vi "EXCEL TRIALS.vi"() -> ()   [LabVIEW 2021]
panel:
  out "PATH OUT":path
  in  "WRITE DATA INPUT":string
  out "READ RESPONSE":string
  in  "Enum":enum16{"READ", "WRITE"}(ring)
  in  "CLOSE/OPEN":bool
  in  "RANGE":string
  in  "Excel._Worksheet":refnum<k7>
  in  "SHEET":string
  in  "Stop":bool
  out "error out":errorcluster
  in  "error in":errorcluster
  in  "Excel._Application":refnum<k7>
  in  "PATH IN":path
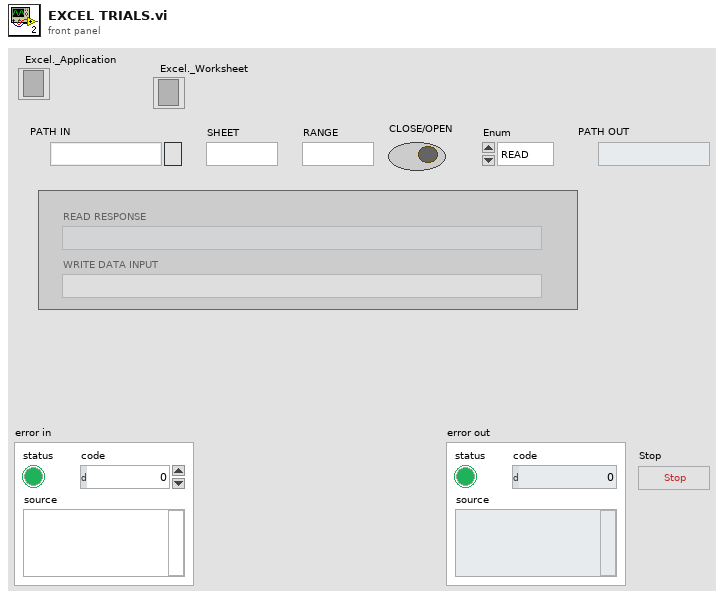
[diagram p1: front panel]
types:
  T1 = enum8{"Enabled", "Disabled", "Disabled and Grayed Out"}
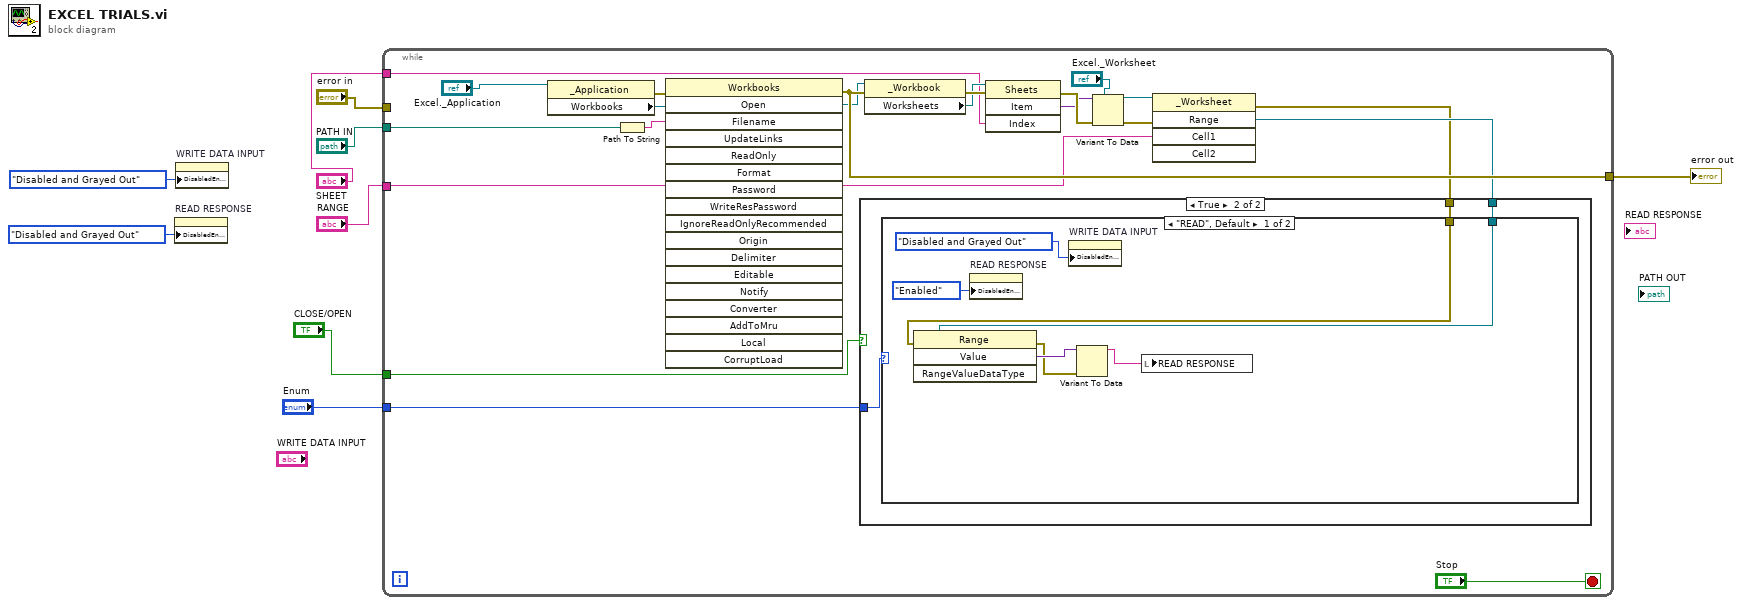
[diagram p0: block diagram]
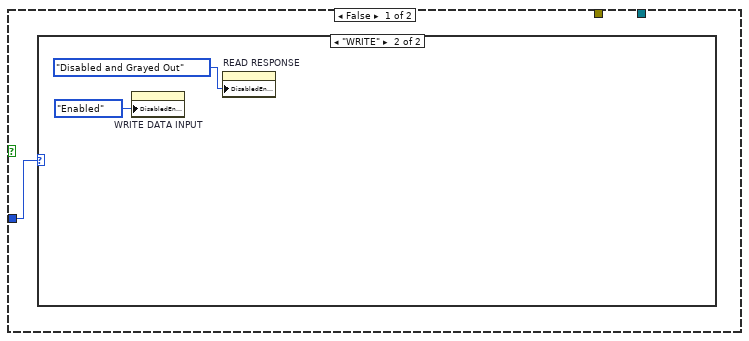
[diagram p2: hidden frame]
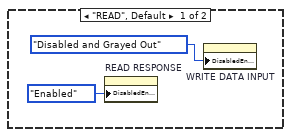
[diagram p3: hidden frame]
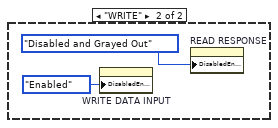
[diagram p4: hidden frame]
diagram:
  n1 = property on="READ RESPONSE" class="Str"("DisabledEnum"=T1."Disabled and Grayed Out" ("Disabled")) -> ()  [unwired: 2 in, 2 out]
  n2 = property on="WRITE DATA INPUT" class="Str"("DisabledEnum"=T1."Disabled and Grayed Out" ("Disabled")) -> ()  [unwired: 2 in, 2 out]
  n3 = while {
    tunnel: "error in" -> [_]
    tunnel: "PATH IN" -> [w27]
    tunnel: [w25] -> w7
    tunnel: "SHEET" -> [w21]
    tunnel: "RANGE" -> [w15]
    tunnel: "CLOSE/OPEN" -> [w14]
    tunnel: "Enum" -> [w13]
    stop <- "Stop" stop-if-true
    n4 = property class="_Application"(reference="Excel._Application") -> (error out=w30:errorcluster, "Workbooks"=w29:refnum<k7>)  [unwired: 1 in, 1 out]
    n5 = Path To String(path=w27) -> (string=w28:string)
    n6 = invoke class="Workbooks" method="Open"(reference=w29, error in=w30, "Filename"=w28) -> (error out=w25:errorcluster, "Open"=w24:refnum<k7>)  [unwired: 15 in, 16 out]
    n7 = property class="_Workbook"(reference=w24, error in=w25) -> (error out=w23:errorcluster, "Worksheets"=w22:refnum<k7>)  [unwired: 1 out]
    n8 = invoke class="Sheets" method="Item"(reference=w22, error in=w23, "Index"=w21) -> (error out=w20:errorcluster, "Item"=w19:variant)  [unwired: 1 in, 2 out]
    n9 = Variant To Data(error in=w20, type="Excel._Worksheet", Variant=w19) -> (data=w16:refnum<k7>, error out=w17:errorcluster)
    n10 = invoke class="_Worksheet" method="Range"(reference=w16, error in=w17, "Cell1"=w15) -> (error out=w11:errorcluster, "Range"=w12:refnum<k7>)  [unwired: 2 in, 3 out]
    n11 = case shown="True" w14 {
      tunnel: w13 -> [w31 w38]
      tunnel: w12 -> [_ w37]
      tunnel: w11 -> [_ w36]
      frame False {
        n12 = case shown="\"WRITE\"" w31 {
          frame "READ", Default {
            n13 = property on="READ RESPONSE" class="Str"("DisabledEnum"=T1."Enabled" ("Disabled")) -> ()  [unwired: 2 in, 2 out]
            n14 = property on="WRITE DATA INPUT" class="Str"("DisabledEnum"=T1."Disabled and Grayed Out" ("Disabled")) -> ()  [unwired: 2 in, 2 out]
          }
          frame "WRITE" {
            n15 = property on="WRITE DATA INPUT" class="Str"("DisabledEnum"=T1."Enabled" ("Disabled")) -> ()  [unwired: 2 in, 2 out]
            n16 = property on="READ RESPONSE" class="Str"("DisabledEnum"=T1."Disabled and Grayed Out" ("Disabled")) -> ()  [unwired: 2 in, 2 out]
          }
        }
      }
      frame True {
        n17 = case shown="\"READ\", Default" w38 {
          tunnel: w37 -> [w43 _]
          tunnel: w36 -> [w39 _]
          frame "READ", Default {
            n18 = invoke class="Range" method="Value"(reference=w43, error in=w39) -> (error out=w40:errorcluster, "Value"=w42:variant)  [unwired: 2 in, 2 out]
            n19 = property on="READ RESPONSE" class="Str"("DisabledEnum"=T1."Enabled" ("Disabled")) -> ()  [unwired: 2 in, 2 out]
            n20 = property on="WRITE DATA INPUT" class="Str"("DisabledEnum"=T1."Disabled and Grayed Out" ("Disabled")) -> ()  [unwired: 2 in, 2 out]
            n21 = Variant To Data(error in=w40, Variant=w42) -> (data=w41:string)  [unwired: 1 in, 1 out]
            n22 = local write "READ RESPONSE"(w41) -> ()
          }
          frame "WRITE" {
            n23 = property on="WRITE DATA INPUT" class="Str"("DisabledEnum"=T1."Enabled" ("Disabled")) -> ()  [unwired: 2 in, 2 out]
            n24 = property on="READ RESPONSE" class="Str"("DisabledEnum"=T1."Disabled and Grayed Out" ("Disabled")) -> ()  [unwired: 2 in, 2 out]
          }
        }
      }
    }
  }
  "error out" <- w7
